vi "Convert Cluster INI String.vi"(8 "error in (no error)":errorcluster, 9 "Indentation String (4-space)":string="    ", 11 "string in":string) -> (0 "error out":errorcluster, 3 "string out":string)   [LabVIEW 2019]
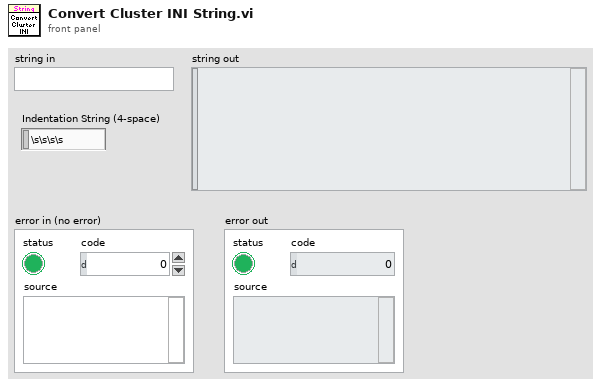
[diagram p1: front panel]
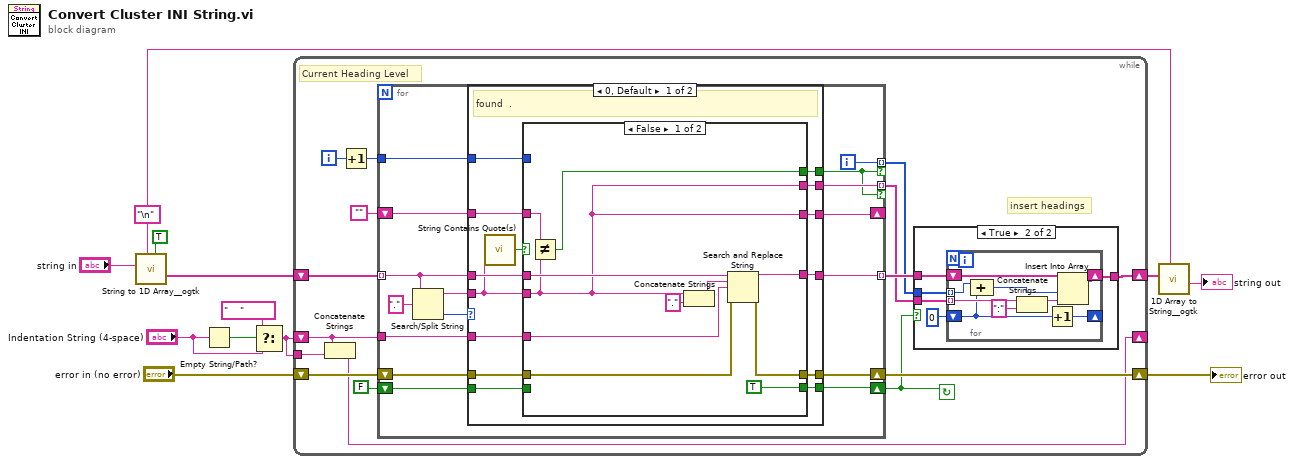
[diagram p0: block diagram]
diagram:
  w8 = "\n"
  n1 = call <userlib>:"String to 1D Array__ogtk.vi"("ignore duplicate delimiters? (F=No)"=TRUE, "delimiter (Tab)"=w8, "string"="string in") -> ("Array of Strings"=w10:string[])  [unwired: 8 in]
  n2 = Empty String/Path?(string/path="Indentation String (4-space)") -> (empty?=w6:bool)
  n3 = Select(t="    ", s=w6, f="Indentation String (4-space)") -> (s? t:f=w1:string)
  n4 = while {
    shift-right: [w22] -> w9
    shift-left: w10 -> [w27]
    shift-right: [w25] -> w3
    shift-left: "error in (no error)" -> [w26]
    shift-right: [w18] -> _
    shift-left: w1 -> [w17]
    tunnel: w1 -> [w16]
    i -> [w15]
    stop <- w19 continue-if-true
    # "Current Heading Level"
    # "insert headings"
    n5 = Concatenate Strings(w17, w16) -> (w18:string)
    n6 = Increment(x=w15) -> (x+1=w14:i32)
    n7 = for {
      tunnel: w27 -> [w53] mode=indexing
      shift-right: [w57] -> _
      shift-left: "" -> [w55]
      tunnel: [w52] -> w21 mode=indexing
      tunnel: w17 -> [w51]
      shift-right: [w49] -> w25
      shift-left: w26 -> [w50]
      shift-right: [w47] -> w19
      shift-left: FALSE -> [w48]
      tunnel: [w46] -> w20 mode=indexing if=w43
      tunnel: w14 -> [w45]
      tunnel: [w44] -> w13 mode=indexing if=w43
      i -> [w46]
      n8 = Search/Split String(string=w53, search string/char (-)=".") -> (substring before match=w56:string, offset of match=w54:i32)  [unwired: 1 in, 1 out]
      n9 = case shown="0, Default" w54 {
        tunnel: [w72 w91] -> w57
        tunnel: w56 -> [w62 _]
        tunnel: w55 -> [w71 w91]
        tunnel: w53 -> [w70 w90]
        tunnel: [w69 w90] -> w52
        tunnel: w51 -> [w68 _]
        tunnel: w50 -> [w67 w89]
        tunnel: [w66 w89] -> w49
        tunnel: w48 -> [w65 w88]
        tunnel: [w64 w88] -> w47
        tunnel: [w63 _] -> w43
        tunnel: w45 -> [w60 _]
        tunnel: [w59 _] -> w44
        frame 0, Default {
          # "found  ."
          n10 = call "String Contains Quote(s).vi"("String"=w62) -> ("Contains quotes?"=w61:bool)  [unwired: 8 in]
          n11 = case shown="False" w61 {
            tunnel: [w75 w87] -> w72
            tunnel: w71 -> [w83 w87]
            tunnel: w70 -> [w82 w86]
            tunnel: [w81 w86] -> w69
            tunnel: w68 -> [w80 _]
            tunnel: w67 -> [w79 w85]
            tunnel: [w78 w85] -> w66
            tunnel: w65 -> [_ w84]
            tunnel: [TRUE w84] -> w64
            tunnel: [w76 _] -> w63
            tunnel: w62 -> [w75 _]
            tunnel: w60 -> [_ _]
            tunnel: [w75 _] -> w59
            frame False {
              n12 = Not Equal?(x=w83, y=w75) -> (x != y?=w76:bool)
              n13 = Concatenate Strings(w75, "." ("string")) -> (w73:string)
              n14 = Search and Replace String(input string=w82, search string=w73, replace string=w80, error in=w79) -> (result string=w81:string, error out=w78:errorcluster)  [unwired: 4 in, 2 out]
            }
            frame True {
              # "This is a decimal number"
            }
          }
        }
        frame -1 {
          # "no . found: leave string as is"
        }
      }
    }
    n15 = case shown="True" w19 {
      tunnel: [w28 w33] -> w22
      tunnel: w21 -> [w28 w32]
      tunnel: w20 -> [_ w31]
      tunnel: w13 -> [_ w30]
      frame False {
      }
      frame True {
        n16 = for {
          tunnel: w31 -> [w40] mode=indexing
          tunnel: w30 -> [w39] mode=indexing
          shift-right: [w42] -> w33
          shift-left: w32 -> [w41]
          shift-right: [w34] -> _
          shift-left: 0 -> [w35]
          n17 = Compound Arithmetic op=ADD(w40, w35) -> (w36:i32)
          n18 = Concatenate Strings(w39, ":" ("string")) -> (w38:string)
          n19 = Increment(x=w35) -> (x+1=w34:i32)
          n20 = Insert Into Array(array=w41, index=w36, new element=w38) -> (w42:string[])
        }
      }
    }
  }
  "error out" <- w3
  n21 = call <userlib>:"1D Array to String__ogtk.vi"("delimiter (Tab)"=w8, "Array of Strings"=w9) -> ("delimited string"=→"string out":string)  [unwired: 9 in]
